vi "Global Log To String.vi"(10 "Log":T1) -> (3 "Log String":string)   [LabVIEW 2020, in "Communicable State Machine.lvlib"]
doc: "<b>Inputs:</b>\n - <b>Log</b>:\n\n<b>Outputs:</b>\n - <b>String</b>:"
uses:
  Communicable State Machine.lvlib
  _CSM_GlobalLog_MSG.ctl
  _CSM_Response Source Message.ctl
  _CSM_GlobalLog_MSG_TYPE.ctl
  CSM - Convert Error to Argument.vi
  CSM - Make String Arguments Safe.vi
  CSM - Keywords.vi
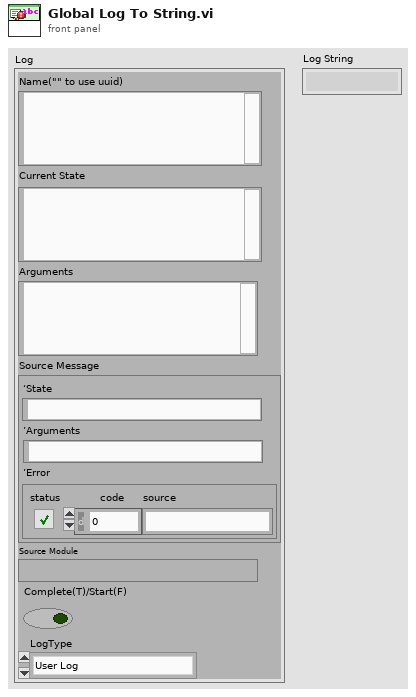
[diagram p1: front panel]
types:
  T1 = typedef "Communicable State Machine.lvlib/_CSM_GlobalLog_MSG.ctl" = cluster{"Name(\"\" to use uuid)":string, "Current State":string, "Arguments":string, "Source Message":T2, "Source Module":string, "Complete(T)/Start(F)":bool, "LogType":T3}
  T2 = typedef "Communicable State Machine.lvlib/_CSM_Response Source Message.ctl" = cluster{"‘State":string, "’Arguments":string, "’Error":errorcluster}
  T3 = typedef "Communicable State Machine.lvlib/_CSM_GlobalLog_MSG_TYPE.ctl" = enum16{"User Log", "State Change", "Status", "Interrupt", "Register", "Unregister", "Error Log", "Module Created", "Module Destroyed"}
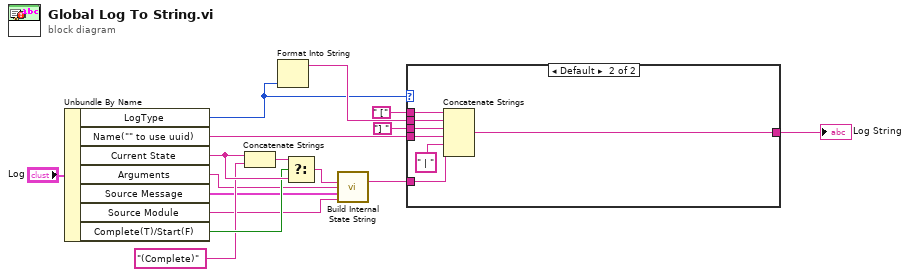
[diagram p0: block diagram]
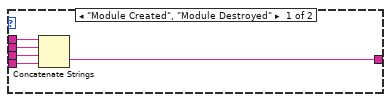
[diagram p2: hidden frame]
diagram:
  n1 = Unbundle By Name("Log") -> ("LogType"=w1:T3, "Name(\"\" to use uuid)"=w4:string, "Current State"=w12:string, "Arguments"=w5:string, "Source Message"=w6:T2, "Source Module"=w7:string, "Complete(T)/Start(F)"=w10:bool)
  n2 = Concatenate Strings(w12, "(Complete)" ("string")) -> (w11:string)
  n3 = Format Into String(w1) -> (resulting string=w16:string)  [unwired: 3 in, 1 out]
  n4 = Select(t=w11, s=w10, f=w12) -> (s? t:f=w13:string)
  n5 = call "Build Internal State String.vi"("State"=w13, "Arguments (\"\")"=w5, ">> Response Source Message >>"=w6, "Source (\"\")"=w7) -> ("State with Arguments"=w9:string)  [unwired: 11 in]
  n6 = case shown="Default" w1 {
    tunnel: w16 -> [w20 w28]
    tunnel: "] " ("string") -> [w19 w27]
    tunnel: " [" ("string") -> [w21 w26]
    tunnel: w4 -> [w18 w23]
    tunnel: [w17 w22] -> w2
    tunnel: w9 -> [_ w24]
    frame "Module Created", "Module Destroyed" {
      n7 = Concatenate Strings(w21, w20, w19, w18) -> (w17:string)
    }
    frame Default {
      n8 = Concatenate Strings(w26, w28, w27, w23, " | " ("string"), w24) -> (w22:string)
    }
  }
  "Log String" <- w2
